vi "linScale.vi"(1 "scale":cluster{"m":dbl, "b":dbl}, 2 "val":sgl) -> (0 "scaled val":dbl)   [LabVIEW 2024]
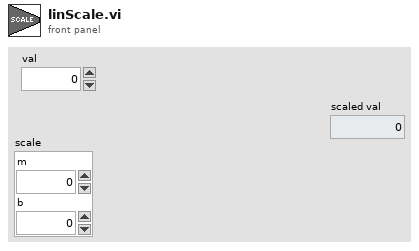
[diagram p1: front panel]
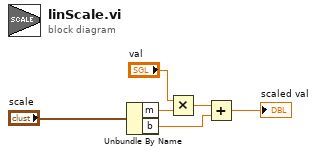
[diagram p0: block diagram]
diagram:
  n1 = Unbundle By Name("scale") -> ("m"=w5:dbl, "b"=w2:dbl)
  n2 = Multiply(x="val", y=w5) -> (x*y=w3:dbl)
  n3 = Add(x=w3, y=w2) -> (x+y=→"scaled val":dbl)
